vi "to boolean.vi"(8 "error in":errorcluster, 11 "byte in":u8) -> (0 "error out":errorcluster, 3 "boolean":bool)   [LabVIEW 2020, in "wamplv.lvlib" / "MessagePack.lvclass"]
uses:
  MessagePack.lvclass
  <vilib>/ErrorRing/Error Ring.xnode
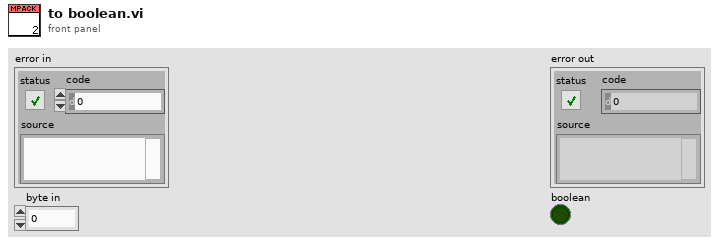
[diagram p1: front panel]
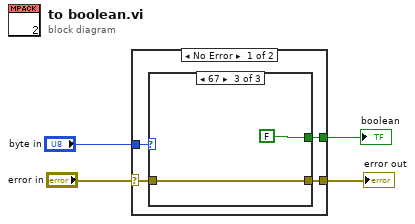
[diagram p0: block diagram]
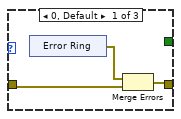
[diagram p2: hidden frame]
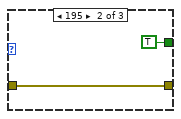
[diagram p3: hidden frame]
diagram:
  n1 = case shown="No Error" "error in" {
    selector: "error in" -> [w7 w17]
    tunnel: "byte in" -> [w8 _]
    tunnel: [w6 w17] -> w2
    tunnel: [w5 _] -> w1
    frame No Error {
      n2 = case shown="67" w8 {
        tunnel: [_ TRUE FALSE] -> w5
        tunnel: w7 -> [w9 w13 w15]
        tunnel: [w11 w13 w15] -> w6
        frame 0, Default {
          n3 = xnode "Error Ring"() -> ("error out"=w10:errorcluster)
          n4 = Merge Errors(w10, w9) -> (w11:errorcluster)
        }
        frame 195 {
        }
        frame 67 {
        }
      }
    }
    frame Error {
    }
  }
  "error out" <- w2
  "boolean" <- w1
